vi "XML-String und Datei vergleichen.vi"(9 "XML-String":string, 10 "Datentypen aus Datei":string[](array[string]), 11 "Namen aus Datei":string[](array[string])) -> (1 "nicht gleich":bool, 2 "Fehler Datentyp":bool, 3 "Fehler Name":bool)   [LabVIEW 2020, in "Anlagenuebersicht.lvlib" / "VisBx Anzeige.lvlib"]
doc: "Vergleicht die Namen und Datentypen aus dem XML-String (Prozessbild aus aktueller Umgebungsvariable) mit den Namen und Datentypen, die aus der TDMS-Datei einer Visualisierung stammen.\n\nBei Unterschieden ist die Prozessvariable nur dann funktionsfähig, wenn neue Elemente im Cluster hinten angefügt wurden. Die neuen Elemente werden dann nicht dargestellt.\n\nMangelnde Übereinstimmung wird gemeldet in\n\"Fehler Name\": Namen stimmen nicht überein\n\"Fehler Datentyp\": Datentypen stimmen nicht überein\n\"nicht gleich\": beide Fälle ODER-verknüpft"
uses:
  VisBx Anzeige.lvlib
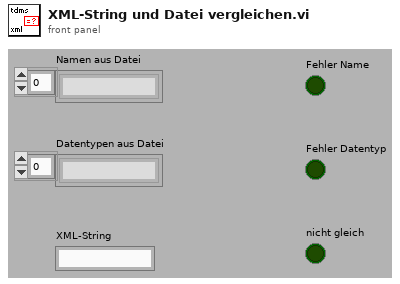
[diagram p1: front panel]
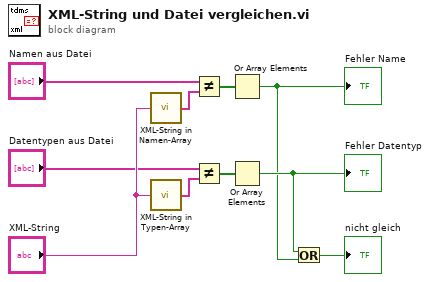
[diagram p0: block diagram]
diagram:
  n1 = call "XML-String in Namen-Array.vi"("XML-String"="XML-String") -> ("Namen (ohne Cluster)"=w9:string[])
  n2 = call "XML-String in Typen-Array.vi"("XML-String"="XML-String") -> ("Typen (ohne Cluster)"=w6:string[])
  n3 = Not Equal?(x="Namen aus Datei", y=w9) -> (x != y?=w5:bool[])
  n4 = Not Equal?(x="Datentypen aus Datei", y=w6) -> (x != y?=w4:bool[])
  n5 = Or Array Elements(Boolean array=w5) -> (logical OR=w2:bool)
  "Fehler Name" <- w2
  n6 = Or Array Elements(Boolean array=w4) -> (logical OR=w3:bool)
  "Fehler Datentyp" <- w3
  n7 = Or(x=w3, y=w2) -> (x .or. y?=→"nicht gleich":bool)
